vi "escribirCSV.vi"(7 "Byte Stream File in":refnum<file>, 8 "error in (no error)":errorcluster, 9 "millisecond timer value in":u32, 10 "datalogger_cluster":T1) -> (0 "error out":errorcluster, 1 "millisecond timer value out":u32, 5 "Byte Stream File out":refnum<file>)   [LabVIEW 2026]
uses:
  Ctrl_Estados.ctl
  Control/Ctrl_EscrituraComandos.ctl
  Control/Ctrl_Errores.ctl
  Control/Ctrl_Motores_Valores.ctl
  Control/Ctrl_datos6motores_final.ctl
  Control/Ctr_Enc_Values.ctl
  Control/Ctrl_Array_Enc_Out_final.ctl
  Control/Ctrl_DataLoggerQueue.ctl
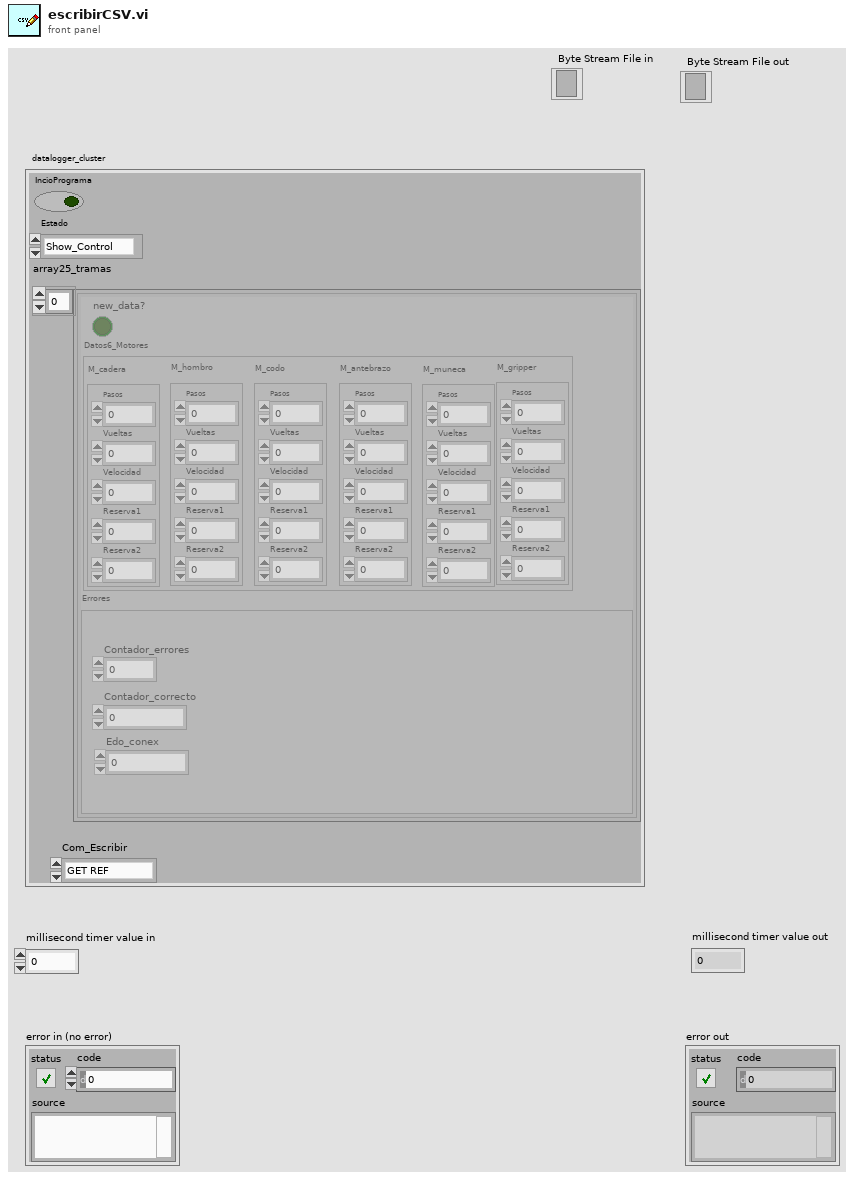
[diagram p1: front panel]
types:
  T1 = typedef "Ctrl_DataLoggerQueue.ctl" = cluster{"IncioPrograma":bool, "Estado":T2, "Com_Escribir":T3, "array25_tramas":T4}
  T2 = typedef "Ctrl_Estados.ctl" = enum16{"Show_Control", "LogData", "Idle", "SHOW PID", "PID_GUI", "Stop", "Show_Dashboard", "Reconnect", "Log_Data_All", "Start", "WRITE_DATA", "SEND_COM"}
  T3 = typedef "Ctrl_EscrituraComandos.ctl" = enum16{"GET REF", "SEND ROUTINE", "MOVE MANUAL", "SEND ESP32", "SET REF"}
  T4 = typedef "Ctrl_Array_Enc_Out_final.ctl" = T5[]
  T5 = typedef "Ctr_Enc_Values.ctl" = cluster{"Datos6_Motores":T6, "Errores":T8, "new_data?":bool}
  T6 = typedef "Ctrl_datos6motores_final.ctl" = cluster{"M_cadera":T7, "M_hombro":T7, "M_codo":T7, "M_antebrazo":T7, "M_muneca":T7, "M_gripper":T7}
  T7 = typedef "Ctrl_Motores_Valores.ctl" = cluster{"Pasos":i32, "Vueltas":i16, "Velocidad":dbl, "Reserva1":u8, "Reserva2":u8}
  T8 = typedef "Ctrl_Errores.ctl" = cluster{"Contador_correcto":u32, "Contador_errores":u32, "Edo_conex":u32}
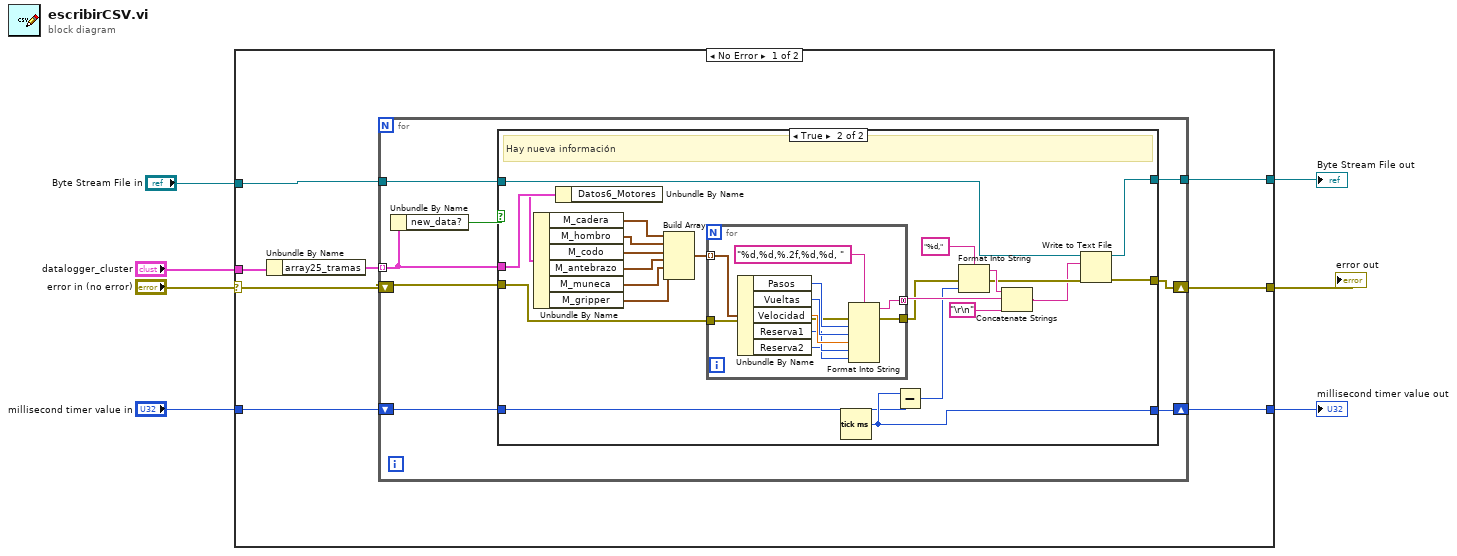
[diagram p0: block diagram]
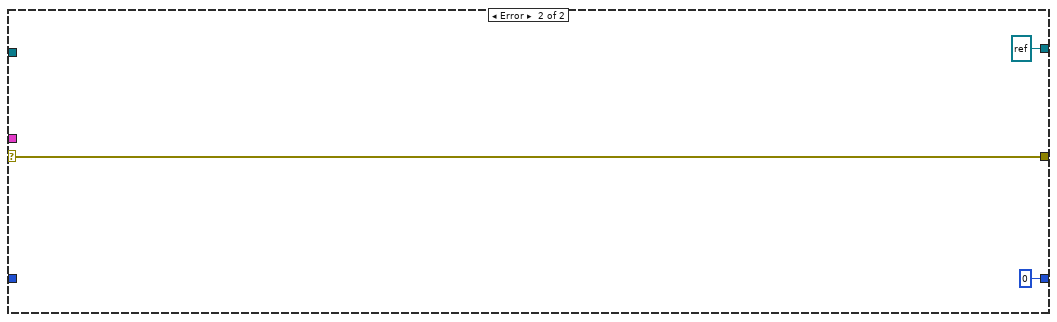
[diagram p3: hidden frame]
diagram:
  n1 = case shown="No Error" "error in (no error)" {
    selector: "error in (no error)" -> [w8 w61]
    tunnel: [w15 refnum<file> refnum ("refnum out")] -> w7
    tunnel: "Byte Stream File in" -> [w14 _]
    tunnel: "datalogger_cluster" -> [w12 _]
    tunnel: "millisecond timer value in" -> [w11 _]
    tunnel: [w10 w61] -> w3
    tunnel: [w9 u32 0 ("millisecond timer value in")] -> w2
    frame No Error {
      n2 = Unbundle By Name(w12) -> ("array25_tramas"=w13:T4)
      n3 = for {
        tunnel: w13 -> [w19] mode=indexing
        shift-right: [w21] -> w10
        shift-left: w8 -> [w22]
        shift-right: [w23] -> w9
        shift-left: w11 -> [w20]
        tunnel: [w17] -> w15
        tunnel: w14 -> [w16]
        n4 = Unbundle By Name(w19) -> ("new_data?"=w18:bool)
        n5 = case shown="True" w18 {
          tunnel: w19 -> [_ w49]
          tunnel: [w25 w40] -> w23
          tunnel: w22 -> [w26 w39]
          tunnel: [w26 w32] -> w21
          tunnel: [w24 w31] -> w17
          tunnel: w20 -> [w25 w30]
          tunnel: w16 -> [w24 w27]
          frame False {
          }
          frame True {
            # "Hay nueva información"
            n6 = Unbundle By Name(w49) -> ("Datos6_Motores"=w48:T6)
            n7 = Unbundle By Name(w48) -> ("M_cadera"=w47:T7, "M_hombro"=w46:T7, "M_codo"=w45:T7, "M_antebrazo"=w44:T7, "M_muneca"=w43:T7, "M_gripper"=w42:T7)
            n8 = Build Array(w47, w46, w45, w44, w43, w42) -> (w41:T7[])
            n9 = for {
              tunnel: w41 -> [w59] mode=indexing
              tunnel: w39 -> [w53]
              tunnel: [w51] -> w38 mode=concatenating
              tunnel: [w50] -> w35
              n10 = Unbundle By Name(w59) -> ("Pasos"=w58:i32, "Vueltas"=w57:i16, "Velocidad"=w56:dbl, "Reserva1"=w55:u8, "Reserva2"=w54:u8)
              n11 = Format Into String(format string="%d,%d,%.2f,%d,%d, ", error in=w53, w58, w57, w56, w55, w54) -> (resulting string=w51:string, error out=w50:errorcluster)  [unwired: 1 in]
            }
            n12 = Tick Count (ms)() -> (millisecond timer value=w40:u32)
            n13 = Subtract(x=w40, y=w30) -> (x-y=w36:u32)
            n14 = Format Into String(format string="%d,", error in=w35, w36) -> (resulting string=w37:string, error out=w33:errorcluster)  [unwired: 1 in]
            n15 = Concatenate Strings(w37, w38, "\r\n") -> (w28:string)
            n16 = Write to Text File(file (use dialog)=w27, text=w28, error in=w33) -> (refnum out=w31:refnum<file>, error out=w32:errorcluster)  [unwired: 1 in, 1 out]
          }
        }
      }
    }
    frame Error {
    }
  }
  "Byte Stream File out" <- w7
  "error out" <- w3
  "millisecond timer value out" <- w2
